vi "Test View No Process Errors Showing and Hiding Panel.vi"(8 "error in (no error)":errorcluster, 11 "UI View Test In":refnum<class "View Test.lvclass">) -> (0 "error out":errorcluster, 3 "UI View Test Out":refnum<class "View Test.lvclass">)   [LabVIEW 2020, in "View Test.lvclass"]
uses:
  View Test.lvclass
  C:/Program Files (x86)/National Instruments/LabVIEW 2020/vi.lib/Astemes/LUnit/Test Case.lvclass
  Mock Error Handler/Mock Error Handler.lvclass
  C:/Git/astemes-triarc-framework/source/Framework/Error Handler Interface/Error Handler Interface.lvclass
  Framework/Process/Process.lvclass/Process.ctl
  Framework/View/View.lvclass/View.ctl
  <vilib>/Astemes/LUnit/Test Case.lvclass/Test Case.ctl
  <vilib>/Astemes/LUnit/LUnit Assertion Result.lvclass/LUnit Assertion Result.ctl
  <vilib>/Astemes/LUnit/LUnit Test Case Result.lvclass/LUnit Test Case Result.ctl
  <vilib>/Astemes/LUnit/LUnit Method Result.lvclass/LUnit Method Result.ctl
  Framework/Process/Protected/Messaging/Enqueue Message.vi
  Framework/Process/Public/Lifecycle/Get Lifecycle State.vi
  Framework/View/Public/Get View VI Reference.vi
  <vilib>/Utility/error.llb/Clear Errors.vi
  Framework/Broadcast Event Helpers/Execution timer.vi
  Framework/Process/Private/SubVIs/Wait for finish.vi
  Framework/Process/Private/SubVIs/Set Lifecycle State.vi
  <vilib>/Astemes/LUnit/Palette/Pass.vi
  <vilib>/Astemes/LUnit/Palette/Fail.vi
  <vilib>/Astemes/LUnit/Set Assertion Type.vi
  Framework/Process/Private/SubVIs/Handle Debug Data.vi
  Framework/Process/Protected/Messaging/Request Message.vi
  <vilib>/Astemes/LUnit/Add test result.vi
  <vilib>/Astemes/LUnit/LUnit Write Passed.vi
  <vilib>/Astemes/LUnit/LUnit Write Message.vi
  <vilib>/Astemes/LUnit/LUnit Write Description.vi
  <vilib>/Astemes/LUnit/LUnit Write Assertion Type.vi
  Framework/Logging/Log Debug.vi
  <vilib>/AdvancedString/1D String Array to Delimited String.vi
  <vilib>/Utility/High Resolution Relative Seconds.vi
  Framework/Process/Private/SubVIs/Enqueue Request Message.vi
  <vilib>/Astemes/LUnit/LUnit Record Assertion Result.vi
  <vilib>/Astemes/LUnit/LUnit Aggregate Assertion Results.vi
  <vilib>/Astemes/LUnit/Assertion Result/LUnit Read Status.vi
  <vilib>/Astemes/LUnit/LUnit Read Message.vi
  <vilib>/Astemes/LUnit/LUnit Read Description.vi
  <vilib>/Astemes/LUnit/Method Result/LUnit Merge Status.vi
  <vilib>/Astemes/LUnit/LUnit Concatenate result strings.vi
  Framework/View/View.lvclass
  C:/Git/astemes-triarc-framework/source/Framework/Process/Process.lvclass
  <vilib>/Utility/error.llb/Error Cluster From Error Code.vi
  Framework/Process/Public/Read Name.vi
  Framework/Process/Private/SubVIs/Wait for Response Message.vi
  Framework/Broadcast Event Helpers/Dequeue Broadcast Message.vi
  <vilib>/Astemes/LUnit/LUnit Assertion Result.lvclass
  Framework/Process/Process.lvclass
  View Test.lvclass/View Test.ctl
  <vilib>/Astemes/LUnit/Test Case.lvclass
  C:/Git/astemes-triarc-framework/source/Framework/Base/Base.lvclass
  C:/Git/astemes-triarc-framework/source/Framework/Logging/Logging.lvclass
  C:/Git/astemes-triarc-framework/source/Framework/View/View.lvclass
  Framework/Broadcast Event Helpers/Broadcast Event Helpers.lvlib
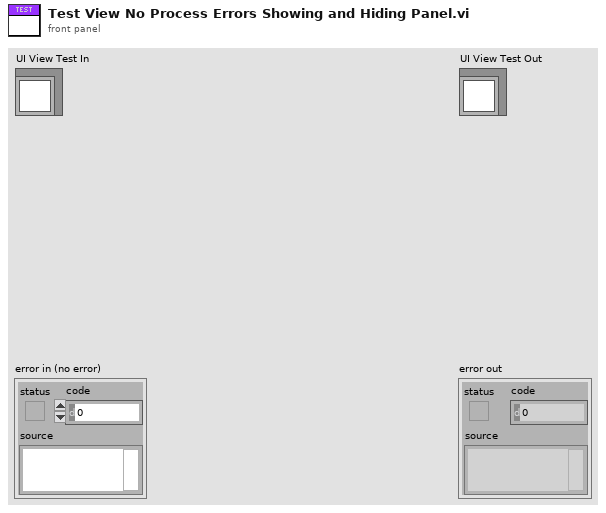
[diagram p1: front panel]
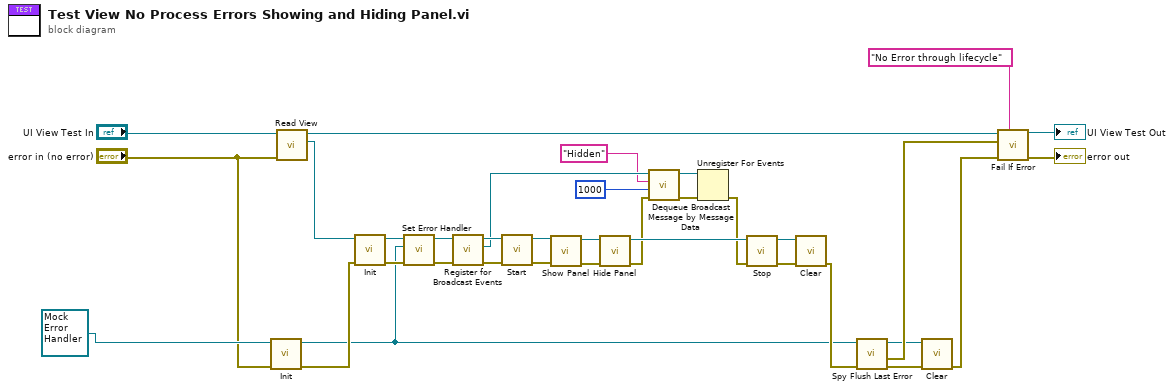
[diagram p0: block diagram]
diagram:
  n1 = call-dynamic "Init.vi"("error in (no error)"="error in (no error)", "Mock Error Handler In"=refnum<class "Mock Error Handler.lvclass"> refnum ("Mock Error Handler.lvclass")) -> ("error out"=w19:errorcluster, "Mock Error Handler Out"=w12:refnum<class "Mock Error Handler.lvclass">)  [unwired: 8 in]
  n2 = call "Read View.vi"("error in (no error)"="error in (no error)", "View Test In"="UI View Test In") -> ("View"=w28:refnum<class "View.lvclass">, "View Test Out"=w33:refnum<class "View Test.lvclass">)  [unwired: 7 in, 1 out]
  n3 = call-dynamic "Init.vi"("error in (no error)"=w19, "View In"=w28) -> ("error out"=w22:errorcluster, "View Out"=w30:refnum<class "View.lvclass">)  [unwired: 8 in]
  n4 = call "Set Error Handler.vi"("error in (no error)"=w22, "Error Handler"=w12, "Process In"=w30) -> ("error out"=w21:errorcluster, "Process Out"=w9:refnum<class "View.lvclass">)  [unwired: 7 in]
  n5 = call "Register for Broadcast Events.vi"("error in (no error)"=w21, "Process In"=w9) -> ("error out"=w10:errorcluster, "Event Registration Refnum Out"=w7:refnum<event-registration>, "Process Out"=w8:refnum<class "View.lvclass">)  [unwired: 7 in]
  n6 = call "Start.vi"("error in (no error)"=w10, "Process In"=w8) -> ("error out"=w26:errorcluster, "Process Out"=w27:refnum<class "View.lvclass">)  [unwired: 7 in, 1 out]
  n7 = call "Show Panel.vi"("error in (no error)"=w26, "View In"=w27) -> ("error out"=w14:errorcluster, "View Out"=w15:refnum<class "View.lvclass">)  [unwired: 8 in]
  n8 = call "Hide Panel.vi"("error in (no error)"=w14, "View In"=w15) -> ("error out"=w3:errorcluster, "View Out"=w29:refnum<class "View.lvclass">)  [unwired: 8 in]
  n9 = call "Dequeue Broadcast Message by Message Data.vi"("error in (no error)"=w3, "Timeout (-1)"=1000, "Message Data"="Hidden" ("Message"), "Event Registration Refnum"=w7) -> ("error out"=w2:errorcluster, "Event Registration Refnum Out"=w1:refnum<event-registration>)  [unwired: 3 in, 3 out]
  n10 = Unregister For Events(event registration refnum=w1, error in=w2) -> (error out=w4:errorcluster)
  n11 = call "Stop.vi"("error in (no error)"=w4, "Process In"=w29) -> ("error out"=w24:errorcluster, "Process Out"=w25:refnum<class "View.lvclass">)  [unwired: 7 in, 1 out]
  n12 = call-dynamic "Clear.vi"("error in (no error)"=w24, "View In"=w25) -> ("error out"=w18:errorcluster)  [unwired: 9 in]
  n13 = call "Spy Flush Last Error.vi"("error in (no error)"=w18, "Mock Error Handler In"=w12) -> ("error out"=w16:errorcluster, "Error"=w13:errorcluster, "Mock Error Handler Out"=w11:refnum<class "Mock Error Handler.lvclass">)  [unwired: 7 in]
  n14 = call-dynamic "Clear.vi"("error in (no error)"=w16, "Mock Process In"=w11) -> ("error out"=w17:errorcluster)  [unwired: 9 in]
  n15 = call <vilib>:"Fail If Error.vi"("Description"="No Error through lifecycle", "error in (no error)"=w17, "Assert error"=w13, "LUnit Test Case In"=w33) -> ("error out"=→"error out":errorcluster, "LUnit Test Case Out"=→"UI View Test Out":refnum<class "View Test.lvclass">)  [unwired: 6 in]
